vi "MFR Flow to SP 2-3.vi"(10 "MFC SPs":dbl[](array[numeric])) -> (2 "MFC array":dbl[](array[numeric]), 4 "SV Array":bool[](array[boolean]))   [LabVIEW 2014]
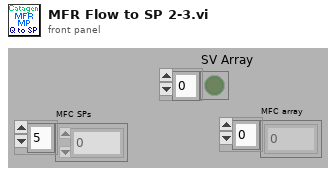
[diagram p1: front panel]
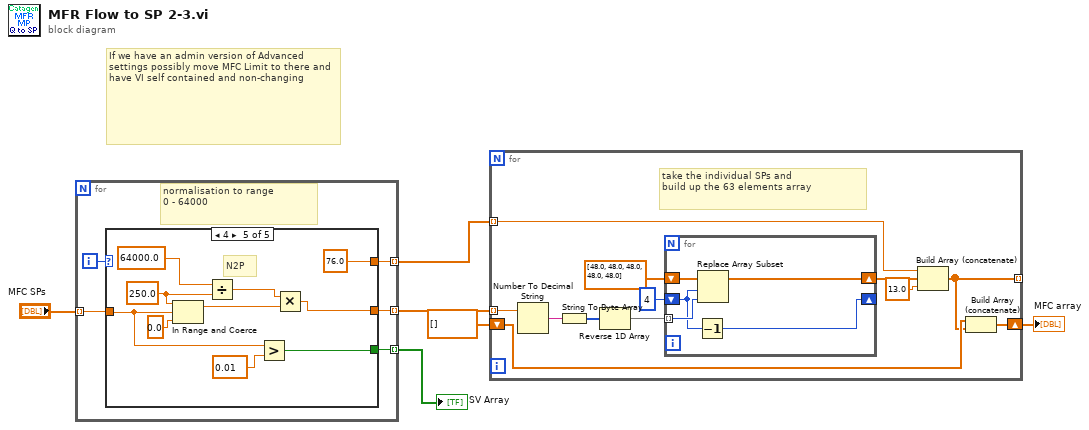
[diagram p0: block diagram]
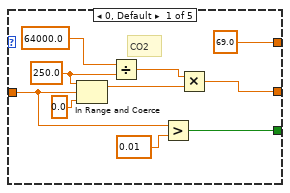
[diagram p2: hidden frame]
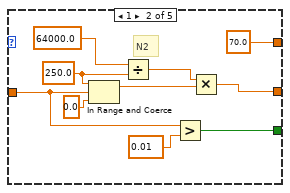
[diagram p3: hidden frame]
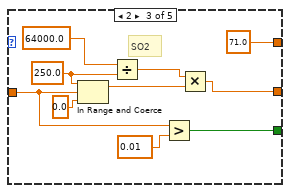
[diagram p4: hidden frame]
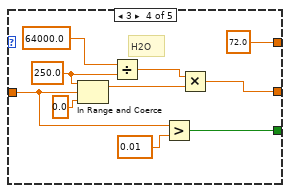
[diagram p5: hidden frame]
diagram:
  # "If we have an admin version of Advanced settings possibly move MFC Limit to there and have VI self contained and non-changing"
  n1 = for {
    tunnel: "MFC SPs" -> [w10] mode=indexing
    tunnel: [w9] -> w3 mode=indexing
    tunnel: [w8] -> w2 mode=indexing
    tunnel: [w7] -> w1 mode=indexing
    i -> [w11]
    # "normalisation to range\n0 - 64000"
    n2 = case shown="4" w11 {
      tunnel: w10 -> [w16 w22 w32 w44 w54]
      tunnel: [w21 w24 w33 w42 w52] -> w9
      tunnel: [69.0 ("y") 70.0 ("y") 71.0 ("y") 72.0 ("y") 76.0 ("y")] -> w8
      tunnel: [w17 w23 w34 w43 w53] -> w7
      frame 0, Default {
        w14 = 250.0 ("upper limit")
        # "CO2"
        n3 = In Range and Coerce(upper limit=w14, x=w16, lower limit=0.0) -> (coerced(x)=w13:dbl)  [unwired: 1 out]
        n4 = Divide(x=64000.0, y=w14) -> (x/y=w12:dbl)
        n5 = Greater?(x=w16, y=0.01) -> (0:w17:bool)
        n6 = Multiply(x=w12, y=w13) -> (x*y=w21:dbl)
      }
      frame 1 {
        w28 = 250.0 ("upper limit")
        # "N2"
        n7 = In Range and Coerce(upper limit=w28, x=w22, lower limit=0.0) -> (coerced(x)=w29:dbl)  [unwired: 1 out]
        n8 = Divide(x=64000.0, y=w28) -> (x/y=w30:dbl)
        n9 = Greater?(x=w22, y=0.01) -> (0:w23:bool)
        n10 = Multiply(x=w30, y=w29) -> (x*y=w24:dbl)
      }
      frame 2 {
        w37 = 250.0 ("upper limit")
        # "SO2"
        n11 = In Range and Coerce(upper limit=w37, x=w32, lower limit=0.0) -> (coerced(x)=w36:dbl)  [unwired: 1 out]
        n12 = Divide(x=64000.0, y=w37) -> (x/y=w35:dbl)
        n13 = Greater?(x=w32, y=0.01) -> (0:w34:bool)
        n14 = Multiply(x=w35, y=w36) -> (x*y=w33:dbl)
      }
      frame 3 {
        w48 = 250.0 ("upper limit")
        # "H2O"
        n15 = In Range and Coerce(upper limit=w48, x=w44, lower limit=0.0) -> (coerced(x)=w49:dbl)  [unwired: 1 out]
        n16 = Divide(x=64000.0, y=w48) -> (x/y=w50:dbl)
        n17 = Greater?(x=w44, y=0.01) -> (0:w43:bool)
        n18 = Multiply(x=w50, y=w49) -> (x*y=w42:dbl)
      }
      frame 4 {
        w58 = 250.0 ("upper limit")
        # "N2P"
        n19 = In Range and Coerce(upper limit=w58, x=w54, lower limit=0.0) -> (coerced(x)=w59:dbl)  [unwired: 1 out]
        n20 = Divide(x=64000.0, y=w58) -> (x/y=w60:dbl)
        n21 = Greater?(x=w54, y=0.01) -> (0:w53:bool)
        n22 = Multiply(x=w60, y=w59) -> (x*y=w52:dbl)
      }
    }
  }
  "SV Array" <- w1
  n23 = for {
    tunnel: w2 -> [w68] mode=indexing
    tunnel: [w64] -> _ mode=indexing
    shift-right: [w63] -> w5
    shift-left: dbl[] [] -> [w65]
    tunnel: w3 -> [w62] mode=indexing
    # "take the individual SPs and \nbuild up the 63 elements array"
    n24 = Number To Decimal String(number=w62) -> (decimal integer string=w69:string)  [unwired: 1 in]
    n25 = String To Byte Array(string=w69) -> (unsigned byte array=w72:u8[])
    n26 = Reverse 1D Array(array=w72) -> (reversed array=w73:u8[])
    n27 = for {
      tunnel: w73 -> [w76] mode=indexing
      shift-right: [w75] -> _
      shift-left: u8 4 -> [w74]
      shift-right: [w77] -> w66
      shift-left: dbl[] [48.0, 48.0, 48.0, 48.0, 48.0] -> [w78]
      n28 = Decrement(x=w74) -> (x-1=w75:u8)
      n29 = Replace Array Subset(array=w78, new element=w76, index=w74) -> (w77:dbl[])
    }
    n30 = Build Array (concatenate)(w68, w66, 13.0) -> (w64:dbl[])
    n31 = Build Array (concatenate)(w65, w64) -> (w63:dbl[])
  }
  "MFC array" <- w5
